vi "Build Byte Stream From G Object.vi"(0 "TwinCAT ADS in":refnum<class "TwinCAT ADS.lvclass">, 5 "Value":variant, 7 "Type Name":string, 9 "Byte Stream in":u8[](array[numeric]), 11 "error in (no error)":errorcluster) -> (4 "TwinCAT ADS out":refnum<class "TwinCAT ADS.lvclass">, 10 "Byte Stream out":u8[](array[numeric]), 15 "error out":errorcluster)   [LabVIEW 2018, in "TwinCAT ADS.lvclass"]
uses:
  TwinCAT ADS.lvclass
  TwinCAT.Ads
  G Primitive to PLC Byte Stream.vi/ebfc1059-5ad7-41af-9a32-6ba056cec1e2.vi
  G Primitive to PLC Byte Stream.vi/6e01a951-886b-41b5-8cd1-fdd71fd1a533.vi
  G Primitive to PLC Byte Stream.vi/09c7a0ef-3209-4624-b801-f77696e71225.vi
  G Primitive to PLC Byte Stream.vi/97b8602c-6a72-408e-90bf-08a26de32539.vi
  G Primitive to PLC Byte Stream.vi/0fd4fbf3-4a18-432c-8f70-6a5c8fef8454.vi
  G Primitive to PLC Byte Stream.vi/afdb5a5e-237c-4be5-828e-15f510cf6cea.vi
  G Primitive to PLC Byte Stream.vi/185a6e12-4d7d-4ad7-9936-0525adb2f85e.vi
  G Primitive to PLC Byte Stream.vi/88229fb8-b58c-494b-bd2b-fea6e0d0ed1b.vi
  G Primitive to PLC Byte Stream.vi/e57df404-389c-41d0-a67c-37c75754ab31.vi
  G Primitive to PLC Byte Stream.vi/d0ee652c-9b86-46ed-9065-57d03aa8de3e.vi
  G Primitive to PLC Byte Stream.vi/886bf0b9-f01c-4a44-b2e2-abccc7b97bfa.vi
  G Primitive to PLC Byte Stream.vi/35f71df7-fc14-4c4d-983c-cf72c138dc9e.vi
  G Primitive to PLC Byte Stream.vi/2d2bc992-a9ff-4dd8-b8fe-74c21cb85899.vi
  G Primitive to PLC Byte Stream.vi/100e4a11-5e4a-45b7-be98-adc9eaebd48d.vi
  G Primitive to PLC Byte Stream.vi/132946d9-68c7-4ade-a66d-dc369520c644.vi
  <vilib>/Utility/error.llb/Trim Whitespace.vi
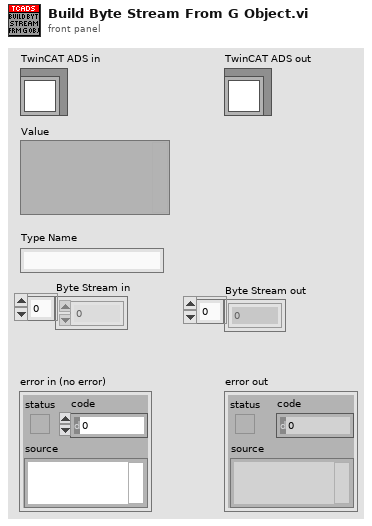
[diagram p1: front panel]
types:
  T1 = typedef "TwinCAT ADS.lvclass/PLC Type.ctl" = enum16{"UNDEFINED", "INT", "DINT", "REAL", "LREAL", "SINT", "BYTE", "UINT", "UDINT", "LINT", "ULINT", "STRING", "WSTRING", "BOOL", "TIME", "LTIME", "DATE", "DT", "TOD", "ARRAY", "JAGGED ARRAY", "STRUCT", "FUNCTION BLOCK", "UNION", "POINTER", "USER DEFINED"}
  T2 = typedef "TwinCAT ADS.lvclass/PLC Sub-Item Type Descriptor.ctl" = cluster{"PLC Type":T1, "Offset":i32, "Byte Size":i32, "[Sub-Item/Array Type Descriptor]":variant[]}
  T3 = typedef "TwinCAT ADS.lvclass/PLC Array Type Descriptor.ctl" = cluster{"Fundamental PLC Type":T1, "Fundamental Type Byte Size":i32, "Item Count":i32, "Dimension Lengths":i32[], "Sub-Item Type Descriptor":variant}
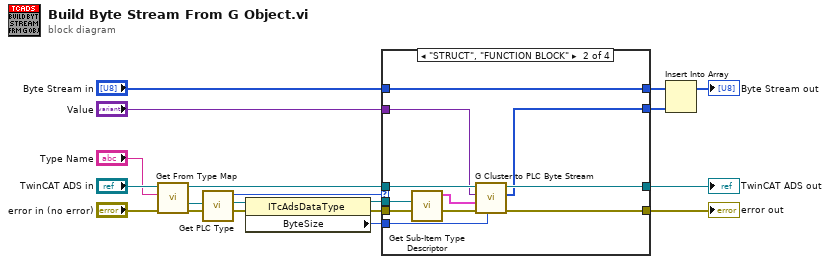
[diagram p0: block diagram]
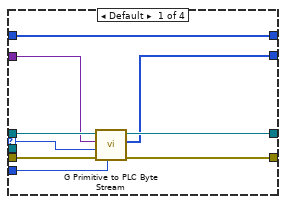
[diagram p2: hidden frame]
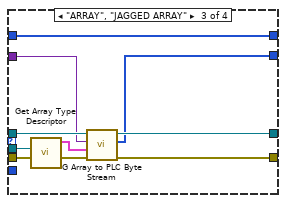
[diagram p3: hidden frame]
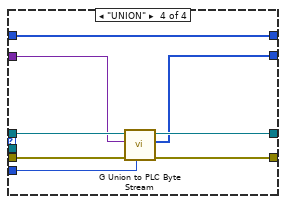
[diagram p4: hidden frame]
diagram:
  n1 = call "Get From Type Map.vi"("error in (no error)"="error in (no error)", "Type Name"="Type Name", "TwinCAT ADS in"="TwinCAT ADS in") -> ("error out"=w12:errorcluster, ".NET AdsDataType"=w11:refnum<k24>, "TwinCAT ADS out"=w16:refnum<class "TwinCAT ADS.lvclass">)  [unwired: 6 in]
  n2 = call "Get PLC Type.vi"("error in (no error)"=w12, ".NET AdsDataType in"=w11) -> ("error out"=w4:errorcluster, ".NET AdsDataType"=w5:refnum<k24>, "PLC Type"=w10:T1)  [unwired: 7 in]
  n3 = property class="ITcAdsDataType"(reference=w5, error in=w4) -> (reference out=w2:refnum<k24>, error out=w3:errorcluster, "ByteSize"=w1:i32)
  n4 = case shown="\"STRUCT\", \"FUNCTION BLOCK\"" w10 {
    selector: w10 -> [w20 _ _ _]
    tunnel: w16 -> [w28 w36 w47 w56]
    tunnel: [w26 w34 w43 w55] -> w15
    tunnel: [w25 w33 w44 w54] -> w14
    tunnel: "Value" -> [w27 w35 w45 w50]
    tunnel: "Byte Stream in" -> [w24 w39 w49 w57]
    tunnel: [w24 w39 w49 w57] -> w8
    tunnel: [w23 w32 w42 w51] -> w7
    tunnel: w3 -> [w22 w31 w41 w53]
    tunnel: w2 -> [_ w30 w40 _]
    tunnel: w1 -> [w21 w29 _ w52]
    frame Default {
      n5 = call "G Primitive to PLC Byte Stream.vi"("Byte Length"=w21, "error in (no error)"=w22, "PLC Type"=w20, "Value"=w27, "TwinCAT ADS in"=w28) -> ("error out"=w25:errorcluster, "Byte Stream"=w23:u8[], "TwinCAT ADS out"=w26:refnum<class "TwinCAT ADS.lvclass">)  [unwired: 4 in]
    }
    frame "STRUCT", "FUNCTION BLOCK" {
      n6 = call "Get Sub-Item Type Descriptor.vi"("error in (no error)"=w31, ".NET AdsDataType"=w30) -> ("error out"=w38:errorcluster, "[Sub-Item Type Descriptor]"=w37:T2[])  [unwired: 7 in, 1 out]
      n7 = call "G Cluster to PLC Byte Stream.vi"("Byte Length"=w29, "error in (no error)"=w38, "[Sub-Item Type Descriptor]"=w37, "Value"=w35, "TwinCAT ADS in"=w36) -> ("error out"=w33:errorcluster, "Byte Stream"=w32:u8[], "TwinCAT ADS out"=w34:refnum<class "TwinCAT ADS.lvclass">)  [unwired: 4 in]
    }
    frame "ARRAY", "JAGGED ARRAY" {
      n8 = call "Get Array Type Descriptor.vi"("error in (no error)"=w41, ".NET AdsDataType"=w40) -> ("error out"=w48:errorcluster, "Array Type Descriptor"=w46:T3)  [unwired: 7 in, 1 out]
      n9 = call "G Array to PLC Byte Stream.vi"("error in (no error)"=w48, "Array Information"=w46, "Value"=w45, "TwinCAT ADS in"=w47) -> ("error out"=w44:errorcluster, "Byte Stream"=w42:u8[], "TwinCAT ADS out"=w43:refnum<class "TwinCAT ADS.lvclass">)  [unwired: 5 in]
    }
    frame "UNION" {
      n10 = call "G Union to PLC Byte Stream.vi"("Byte Length"=w52, "error in (no error)"=w53, "Value"=w50, "TwinCAT ADS in"=w56) -> ("error out"=w54:errorcluster, "Byte Stream"=w51:u8[], "TwinCAT ADS out"=w55:refnum<class "TwinCAT ADS.lvclass">)  [unwired: 5 in]
    }
  }
  "error out" <- w14
  "TwinCAT ADS out" <- w15
  n11 = Insert Into Array(array=w8, new element=w7) -> (→"Byte Stream out":u8[])  [unwired: 1 in]
